vi "LaunchTableLogger.vi"(8 "error in (no error)":errorcluster, 9 "Data Cluster (for Headers)":variant, 10 "TableLogger Config":T1={"TableLogger"=enum."SQLite Logger", "DB File Path"=path "DB.db", "DB Backup Config"={"Directory"=path "DB/Backup", "UTC Time Format"=FALSE, "On Launch"=FALSE, "Interval (Hours)"=100.0, "Size Multiples (Bytes)"=24}}, 11 "Parent Actor In (Unwired if root actor)":refnum<class "Actor.lvclass">) -> (0 "error out":errorcluster, 2 "TableLogger Actor's Enqueuer":refnum<class "Message Enqueuer.lvclass">, 3 "Parent Actor Out":refnum<class "Actor.lvclass">, 5 "object out":refnum<class "TableLogger_Actor.lvclass">)   [LabVIEW 2014, in "TableLogger_Actor.lvlib" / "TableLogger_Actor.lvclass"]
uses:
  TableLogger_Actor.lvclass
  <vilib>/ActorFramework/Actor/Actor.lvclass
  <vilib>/ActorFramework/Message Enqueuer/Message Enqueuer.lvclass
  TableLoggerConfig.ctl
  TableLoggerTypes.ctl
  TableLoggerBackupConfig.ctl
  TableLogger_CSV_Actor/TableLogger_CSV_Actor/TableLogger_CSV_Actor.lvclass
  TableLogger_SQLite_Actor/TableLogger_SQLite_Actor/TableLogger_SQLite_Actor.lvclass
  TableLogger_Actor.lvclass/TableLogger_Actor.ctl
  <vilib>/ActorFramework/Message Enqueuer/Message Enqueuer.lvclass/Message Enqueuer.ctl
  <vilib>/ActorFramework/Message Enqueuer/Enqueue.vi
  <vilib>/ActorFramework/Message Priority Queue/Priority Enqueue.vi
  TableLogger_Actor Messages/BackupDB Msg/BackupDB Msg.lvclass
  TableLogger_Actor.lvlib
panel:
  # "Connector Pane"
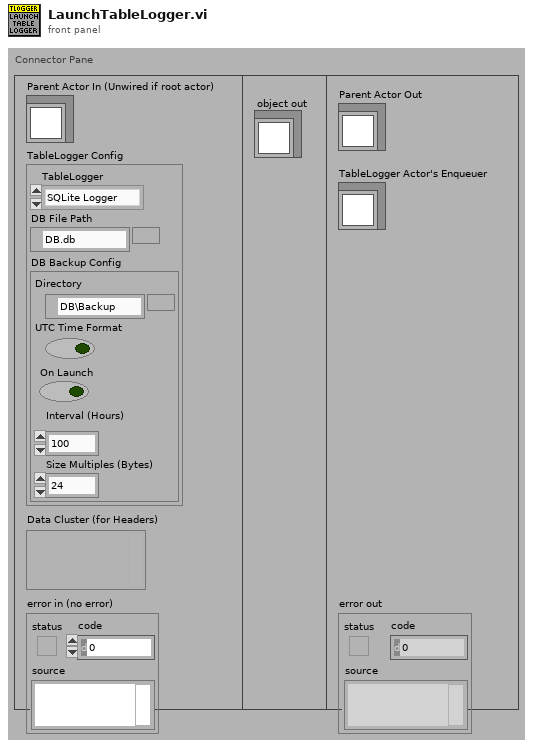
[diagram p1: front panel]
types:
  T1 = typedef "TableLogger_Actor.lvlib/TableLoggerConfig.ctl" = cluster{"TableLogger":T2, "DB File Path":path, "DB Backup Config":T3}
  T2 = typedef "TableLogger_Actor.lvlib/TableLoggerTypes.ctl" = enum16{"CSV Logger", "SQLite Logger"}
  T3 = typedef "TableLogger_Actor.lvlib/TableLoggerBackupConfig.ctl" = cluster{"Directory":path, "UTC Time Format":bool, "On Launch":bool, "Interval (Hours)":dbl, "Size Multiples (Bytes)":i32}
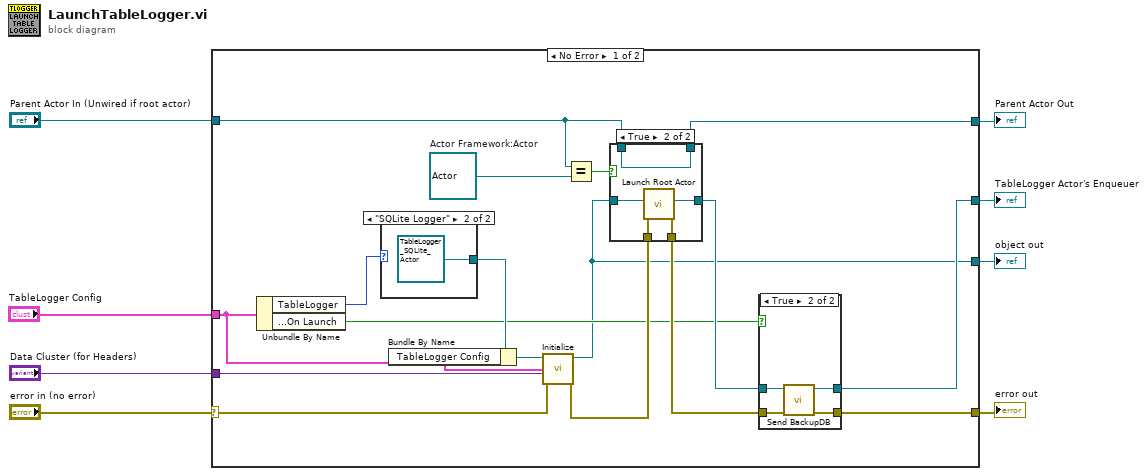
[diagram p0: block diagram]
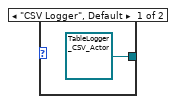
[diagram p3: hidden frame]
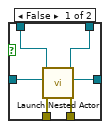
[diagram p4: hidden frame]
diagram:
  n1 = case shown="No Error" "error in (no error)" {
    selector: "error in (no error)" -> [w21 w46]
    tunnel: [w17 w46] -> w7
    tunnel: [w12 _] -> w2
    tunnel: "Parent Actor In (Unwired if root actor)" -> [w19 w45]
    tunnel: "TableLogger Config" -> [w10 _]
    tunnel: "Data Cluster (for Headers)" -> [w20 _]
    tunnel: [w11 w45] -> w4
    tunnel: [w14 _] -> w3
    frame No Error {
      w25 = refnum<class "Actor.lvclass"> refnum  # Actor Framework:Actor
      n2 = Unbundle By Name(w10) -> ("TableLogger"=w23:T2, "DB Backup Config.On Launch"=w13:bool)
      n3 = case shown="\"SQLite Logger\"" w23 {
        tunnel: [refnum<class "TableLogger_CSV_Actor.lvclass"> refnum ("TableLogger_CSV_Actor.lvlib:TableLogger_CSV_Actor.lvclass") refnum<class "TableLogger_SQLite_Actor.lvclass"> refnum ("TableLogger_SQLite_Actor.lvlib:TableLogger_SQLite_Actor.lvclass")] -> w22
        frame "CSV Logger", Default {
        }
        frame "SQLite Logger" {
        }
      }
      n4 = Bundle By Name(cluster=w22, "TableLogger Config"=w10) -> (w9:refnum<class "TableLogger_Actor.lvclass">)
      n5 = call-dynamic "Initialize.vi"("error in (no error)"=w21, "Data Cluster (for Headers)"=w20, "TableLogger Config"=w10, "object in"=w9) -> ("error out"=w18:errorcluster, "object out"=w12:refnum<class "TableLogger_Actor.lvclass">)  [unwired: 6 in]
      n6 = Equal?(x=w19, y=w25) -> (x = y?=w24:bool)
      n7 = case shown="True" w24 {
        tunnel: w19 -> [w39 w44]
        tunnel: [w38 w44] -> w11
        tunnel: w12 -> [w35 w43]
        tunnel: w18 -> [w37 w42]
        tunnel: [w36 w41] -> w16
        tunnel: [w34 w40] -> w15
        frame False {
          n8 = call <vilib>:"Launch Nested Actor.vi"("error in (no error)"=w37, "Nested Actor"=w35, "Caller Actor in"=w39) -> ("error out"=w36:errorcluster, "Nested Actor's Enqueuer"=w34:refnum<class "Message Enqueuer.lvclass">, "Caller Actor out"=w38:refnum<class "Actor.lvclass">)  [unwired: 6 in]
        }
        frame True {
          n9 = call <vilib>:"Launch Root Actor.vi"("error in (no error)"=w42, "Actor"=w43) -> ("error out"=w41:errorcluster, "Actor's Enqueuer"=w40:refnum<class "Message Enqueuer.lvclass">)  [unwired: 8 in]
        }
      }
      n10 = case shown="True" w13 {
        tunnel: [w26 w30] -> w17
        tunnel: w16 -> [w26 w31]
        tunnel: w15 -> [w27 w29]
        tunnel: [w27 w28] -> w14
        frame False {
        }
        frame True {
          n11 = call "Send BackupDB.vi"("error in (no error)"=w31, "Message Enqueuer"=w29) -> ("error out"=w30:errorcluster, "Message Enqueuer out"=w28:refnum<class "Message Enqueuer.lvclass">)  [unwired: 8 in]
        }
      }
    }
    frame Error {
    }
  }
  "error out" <- w7
  "object out" <- w2
  "Parent Actor Out" <- w4
  "TableLogger Actor's Enqueuer" <- w3
